vi "getHardwareInfo.vi"(8 "error in (no error)":errorcluster, 11 "Electrometer in":refnum<class "Electrometer.lvclass">) -> (0 "error out":errorcluster, 2 "electrometerInfo":string, 3 "Electrometer out":refnum<class "Electrometer.lvclass">)   [LabVIEW 2016, in "Electrometer.lvclass"]
uses:
  Electrometer.lvclass
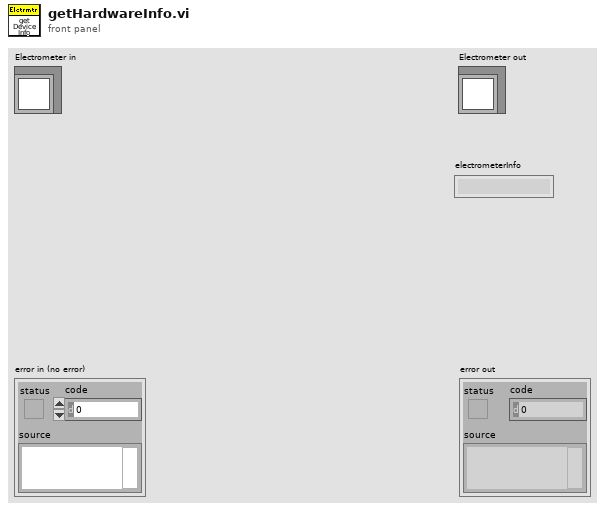
[diagram p1: front panel]
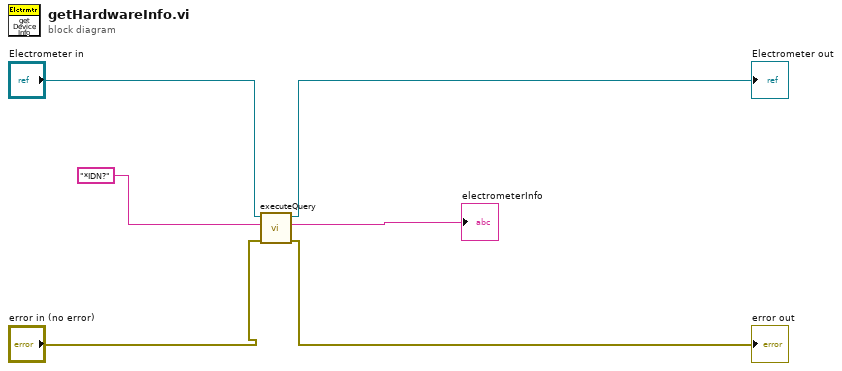
[diagram p0: block diagram]
diagram:
  n1 = call "executeQuery.vi"("error in (no error)"="error in (no error)", "command"="*IDN?", "Electrometer in"="Electrometer in") -> ("error out"=→"error out":errorcluster, "result"=→"electrometerInfo":string, "Electrometer out"=→"Electrometer out":refnum<class "Electrometer.lvclass">)  [unwired: 6 in]
